vi "CIRCLE_v1.vi"(0 "Center-X":i32, 1 "Center-Y":i32, 2 "Angle":i16, 3 "Speed":i32, 4 "Current (mA)":dbl=30.0, 5 "Motor GPIB":u8=6, 6 "Laser GPIB":u8=10) -> ()   [LabVIEW 2010]
uses:
  <vilib>/express/express arith-compare/Formula/XNode/ExpressFormulaBlockNode.xnode
panel:
  out "Quadrant":string
  out "Offset":dbl
  out "Resolution":u16
  out "Radius":u32
  out "Quadrant":u8
  out "dX":i32
  out "dY":i32
  out "Y0":i32
  out "X0":i32
  # "Command description:"
  # "CIRCLE<space>[Displacement to Center Point]:[Curve Displacement Angle]<space>[Speed]<space>[Current]"
  # "User inputs"
  # "Addresses"
  # "Non essential output (for troubleshooting)"
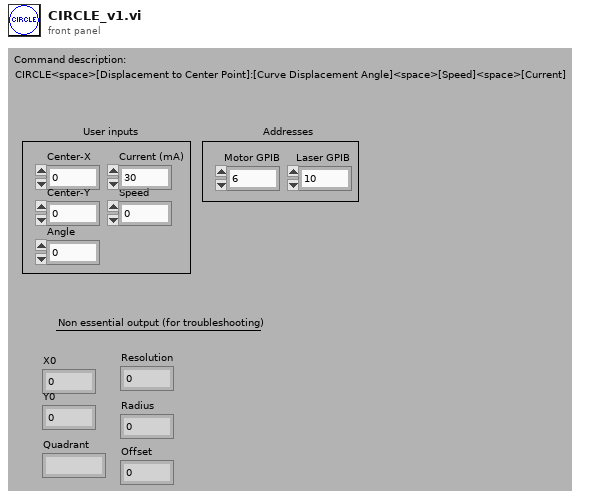
[diagram p1: front panel]
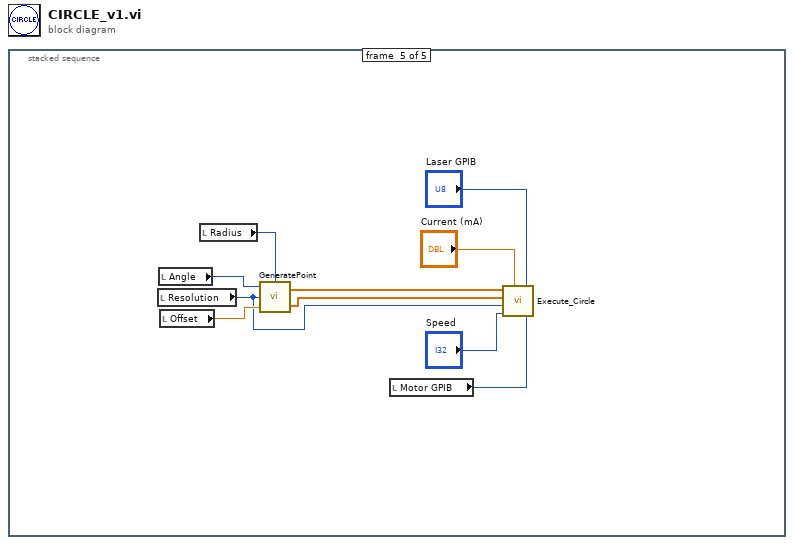
[diagram p0: block diagram]
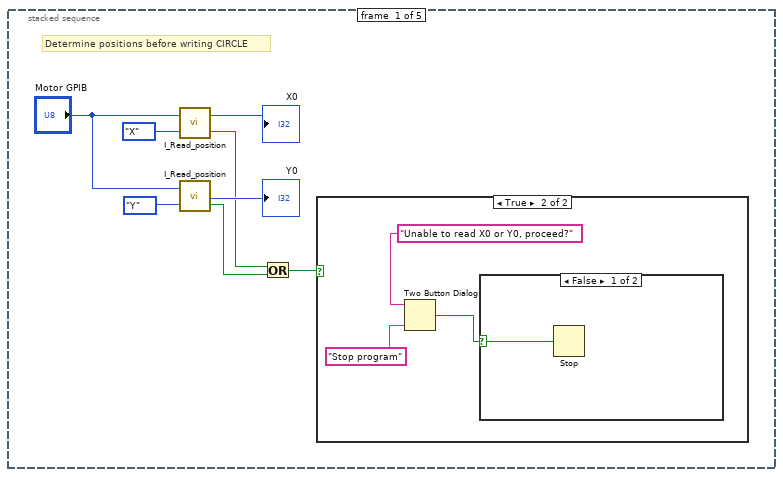
[diagram p2: hidden frame]
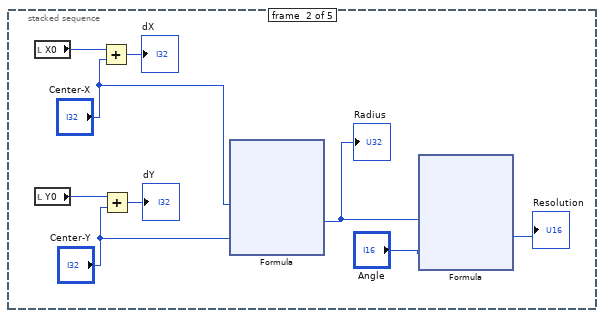
[diagram p5: hidden frame]
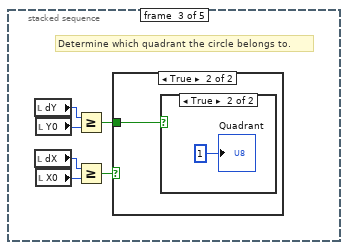
[diagram p6: hidden frame]
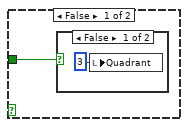
[diagram p7: hidden frame]
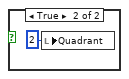
[diagram p8: hidden frame]
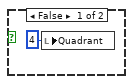
[diagram p9: hidden frame]
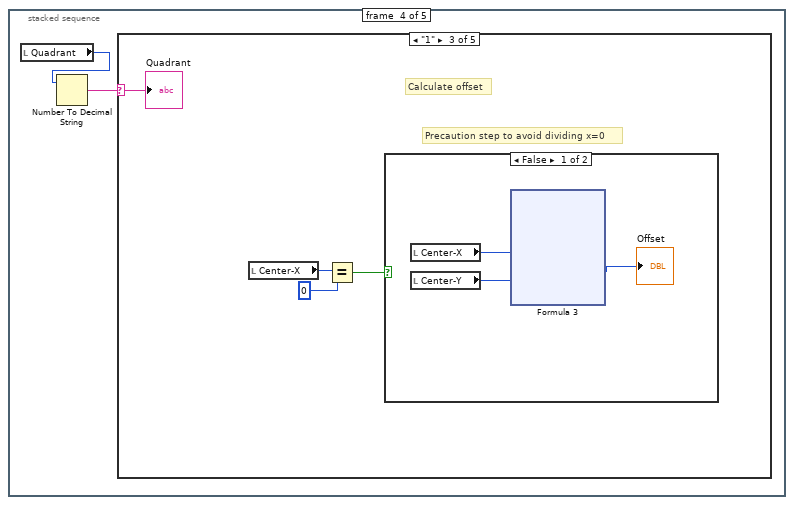
[diagram p10: hidden frame]
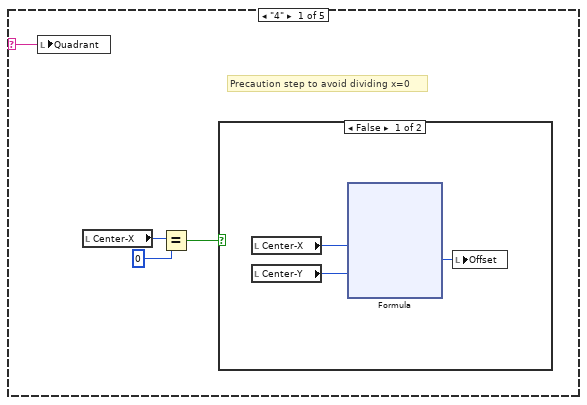
[diagram p11: hidden frame]
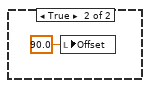
[diagram p12: hidden frame]
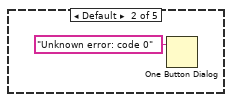
[diagram p13: hidden frame]
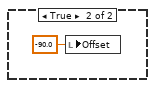
[diagram p14: hidden frame]
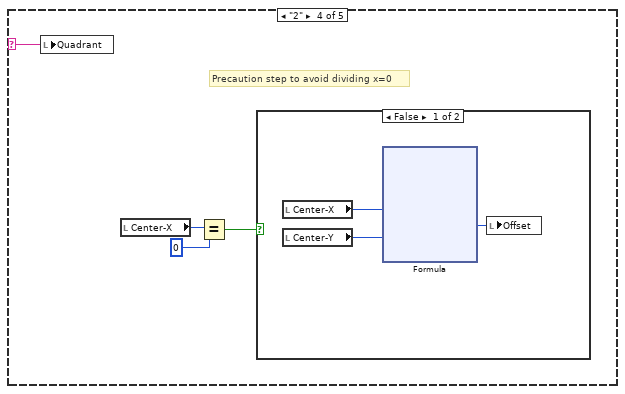
[diagram p15: hidden frame]
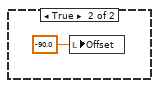
[diagram p16: hidden frame]
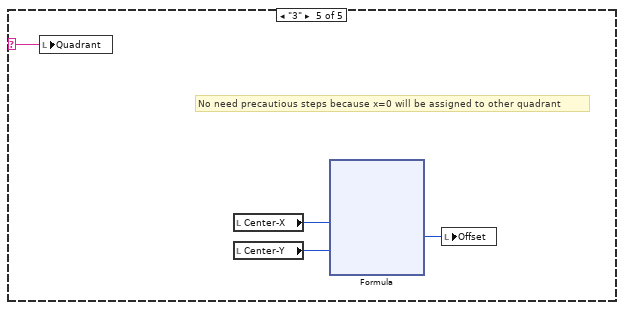
[diagram p17: hidden frame]
diagram:
  n1 = stacked-sequence {
    frame #0 {
      # "Determine positions before writing CIRCLE"
      n2 = call "I_Read_position.vi"("Axis"=enum16{"X", "Y", "Z", "U", "V", "W"}."X", "Motor GPIB"="Motor GPIB") -> ("Error?"=w3:bool, "Position"=→"X0":i32)
      n3 = call "I_Read_position.vi"("Axis"=enum16{"X", "Y", "Z", "U", "V", "W"}."Y", "Motor GPIB"="Motor GPIB") -> ("Error?"=w2:bool, "Position"=→"Y0":i32)
      n4 = Or(x=w3, y=w2) -> (x .or. y?=w1:bool)
      n5 = case shown="True" w1 {
        frame False {
        }
        frame True {
          n6 = Two Button Dialog(message="Unable to read X0 or Y0, proceed?", 1:"Stop program" ("F button name (\"Cancel\")")) -> (T button?=w9:bool)  [unwired: 1 in]
          n7 = case shown="False" w9 {
            selector: w9 -> [w12 _]
            frame False {
              n8 = Stop(stop? (T)=w12) -> ()
            }
            frame True {
            }
          }
        }
      }
    }
    frame #1 {
      n9 = local read "X0"() -> (w14:i32)
      n10 = local read "Y0"() -> (w13:i32)
      n11 = Add(x=w14, y="Center-X") -> (x+y=→"dX":i32)
      n12 = Add(x=w13, y="Center-Y") -> (x+y=→"dY":i32)
      n13 = xnode "Formula"("X1"="Center-X", "X2"="Center-Y") -> ("Result"=w19:i32)  [unwired: 1 in, 1 out]
      "Radius" <- w19
      n14 = xnode "Formula"("X1"=w19, "X2"="Angle") -> ("Result"=→"Resolution":i32)  [unwired: 1 in, 1 out]
    }
    frame #2 {
      # "Determine which quadrant the circle belongs to."
      n15 = local read "dY"() -> (w45:i32)
      n16 = local read "dX"() -> (w47:i32)
      n17 = local read "Y0"() -> (w44:i32)
      n18 = local read "X0"() -> (w46:i32)
      n19 = Greater Or Equal?(x=w45, y=w44) -> (x >= y?=w43:bool)
      n20 = Greater Or Equal?(x=w47, y=w46) -> (x >= y?=w42:bool)
      n21 = case shown="True" w42 {
        tunnel: w43 -> [w48 w51]
        frame False {
          n22 = case shown="False" w48 {
            frame False {
              n23 = local write "Quadrant"(u8 3 ("Dummy")) -> ()
            }
            frame True {
              n24 = local write "Quadrant"(u8 2 ("Dummy")) -> ()
            }
          }
        }
        frame True {
          n25 = case shown="True" w51 {
            frame False {
              n26 = local write "Quadrant"(u8 4 ("Dummy")) -> ()
            }
            frame True {
              "Quadrant" <- u8 1 ("Dummy")
            }
          }
        }
      }
    }
    frame #3 {
      n27 = local read "Quadrant"() -> (w55:u8)
      n28 = Number To Decimal String(number=w55) -> (decimal integer string=w54:string)  [unwired: 1 in]
      n29 = case shown="\"1\"" w54 {
        selector: w54 -> [w56 _ w78 w96 w111]
        frame "4" {
          # "Precaution step to avoid dividing x=0"
          n30 = local write "Quadrant"(w56) -> ()
          n31 = local read "Center-X"() -> (w59:i32)
          n32 = Equal?(x=w59, y=0) -> (x = y?=w57:bool)
          n33 = case shown="False" w57 {
            frame False {
              n34 = local read "Center-X"() -> (w62:i32)
              n35 = local read "Center-Y"() -> (w61:i32)
              n36 = xnode "Formula"("X1"=w62, "X2"=w61) -> ("Result"=w60:i32)  [unwired: 1 in, 1 out]
              n37 = local write "Offset"(w60) -> ()
            }
            frame True {
              n38 = local write "Offset"(90.0 ("Offset")) -> ()
            }
          }
        }
        frame Default {
          n39 = One Button Dialog(message="Unknown error: code 0") -> ()  [unwired: 1 in, 1 out]
        }
        frame "1" {
          # "Calculate offset"
          # "Precaution step to avoid dividing x=0"
          n40 = local read "Center-X"() -> (w77:i32)
          n41 = Equal?(x=w77, y=0) -> (x = y?=w75:bool)
          n42 = case shown="False" w75 {
            frame False {
              n43 = local read "Center-X"() -> (w81:i32)
              n44 = local read "Center-Y"() -> (w80:i32)
              n45 = xnode "Formula 3"("X1"=w81, "X2"=w80) -> ("Result"=→"Offset":i32)  [unwired: 1 in, 1 out]
            }
            frame True {
              n46 = local write "Offset"(-90.0 ("Offset")) -> ()
            }
          }
          "Quadrant" <- w78
        }
        frame "2" {
          # "Precaution step to avoid dividing x=0"
          n47 = local write "Quadrant"(w96) -> ()
          n48 = local read "Center-X"() -> (w95:i32)
          n49 = Equal?(x=w95, y=0) -> (x = y?=w93:bool)
          n50 = case shown="False" w93 {
            frame False {
              n51 = local read "Center-X"() -> (w99:i32)
              n52 = local read "Center-Y"() -> (w98:i32)
              n53 = xnode "Formula"("X1"=w99, "X2"=w98) -> ("Result"=w97:i32)  [unwired: 1 in, 1 out]
              n54 = local write "Offset"(w97) -> ()
            }
            frame True {
              n55 = local write "Offset"(-90.0 ("Offset")) -> ()
            }
          }
        }
        frame "3" {
          # "No need precautious steps because x=0 will be assigned to other quadrant"
          n56 = local write "Quadrant"(w111) -> ()
          n57 = local read "Center-X"() -> (w114:i32)
          n58 = local read "Center-Y"() -> (w113:i32)
          n59 = xnode "Formula"("X1"=w114, "X2"=w113) -> ("Result"=w112:i32)  [unwired: 1 in, 1 out]
          n60 = local write "Offset"(w112) -> ()
        }
      }
    }
    frame #4 {
      n61 = local read "Resolution"() -> (w128:u16)
      n62 = local read "Angle"() -> (w134:i16)
      n63 = local read "Offset"() -> (w133:dbl)
      n64 = local read "Radius"() -> (w132:u32)
      n65 = call "GeneratePoint.vi"("Radius"=w132, "Offset"=w133, "Resolution"=w128, "Angle"=w134) -> ("y-disp"=w130:sgl[], "x-disp"=w131:sgl[])
      n66 = local read "Motor GPIB"() -> (w126:u8)
      n67 = call "Execute_Circle.vi"("x-disp inp."=w131, "y-disp inp."=w130, "Resolution"=w128, "Speed"="Speed", "Current (mA)"="Current (mA)", "Laser GPIB"="Laser GPIB", "Motor GPIB"=w126) -> ()
    }
  }
